vi "LJM logger fill channel setup lists to size.vi"(1 "Default Channel Setup":T1={"Name"=["AIN0", "AIN1", "AIN2", "AIN3", "AIN4", "AIN5", "AIN6", "AIN7", "AIN8", "AIN9", "AIN10", "AIN11", "AIN12", "AIN13", "AIN14", "AIN15", "AIN16", "AIN17", "AIN18", "AIN19", "AIN20", "AIN21", "AIN22", "AIN23", "AIN24", "AIN25", "AIN26", "AIN27", "AIN28", "AIN29", "AIN30", "AIN31", "AIN32", "AIN33", "AIN34", "AIN35", "AIN36", "AIN37", "AIN38", "AIN39", "AIN40", "AIN41", "AIN42", "AIN43", "AIN44", "AIN45", "AIN46", "AIN47", "AIN48", "AIN49", "AIN50", "AIN51", "AIN52", "AIN53", "AIN54", "AIN55", "AIN56", "AIN57", "AIN58", "AIN59", "AIN60", "AIN61", "AIN62", "AIN63", "AIN64", "AIN65", "AIN66", "AIN67", "AIN68", "AIN69", "AIN70", "AIN71", "AIN72", "AIN73", "AIN74", "AIN75", "AIN76", "AIN77", "AIN78", "AIN79", "AIN80", "AIN81", "AIN82", "AIN83", "AIN84", "AIN85", "AIN86", "AIN87", "AIN88", "AIN89", "AIN90", "AIN91", "AIN92", "AIN93", "AIN94", "AIN95", "AIN96", "AIN97", "AIN98", "AIN99"], "", "Scaling Equation"=["y=a", "y=b", "y=c", "y=d", "y=e", "y=f", "y=g", "y=h", "y=i", "y=j", "y=k", "y=l", "y=m", "y=n", "y=o", "y=p", "y=q", "y=r", "y=s", "y=t", "y=u", "y=v", "y=w", "y=x", "y=y", "y=z", "y=a2", "y=b2", "y=c2", "y=d2", "y=e2", "y=f2", "y=g2", "y=h2", "y=i2", "y=j2", "y=k2", "y=l2", "y=m2", "y=n2", "y=o2", "y=p2", "y=q2", "y=r2", "y=s2", "y=t2", "y=u2", "y=v2", "y=w2", "y=x2", "y=y2", "y=z2", "y=a3", "y=b3", "y=c3", "y=d3", "y=e3", "y=f3", "y=g3", "y=h3", "y=i3", "y=j3", "y=k3", "y=l3", "y=m3", "y=n3", "y=o3", "y=p3", "y=q3", "y=r3", "y=s3", "y=t3", "y=u3", "y=v3", "y=w3", "y=x3", "y=y3", "y=z3", "y=a4", "y=b4", "y=c4", "y=d4", "y=e4", "y=f4", "y=g4", "y=h4", "y=i4", "y=j4", "y=k4", "y=l4", "y=m4", "y=n4", "y=o4", "y=p4", "y=q4", "y=r4", "y=s4", "y=t4", "y=u4", "y=v4"], "", "Graph?"=[TRUE, TRUE, TRUE, TRUE, FALSE, FALSE, FALSE, FALSE, FALSE, FALSE, FALSE, FALSE, FALSE, FALSE, FALSE, FALSE]}, 2 "Channel Setup In":T1={"Name"=["AIN0", "AIN1", "AIN2", "AIN3", "AIN4", "AIN5", "AIN6", "AIN7", "AIN8", "AIN9", "AIN10", "AIN11", "AIN12", "AIN13", "AIN14", "AIN15", "AIN16", "AIN17", "AIN18", "AIN19", "AIN20", "AIN21", "AIN22", "AIN23", "AIN24", "AIN25", "AIN26", "AIN27", "AIN28", "AIN29", "AIN30", "AIN31", "AIN32", "AIN33", "AIN34", "AIN35", "AIN36", "AIN37", "AIN38", "AIN39", "AIN40", "AIN41", "AIN42", "AIN43", "AIN44", "AIN45", "AIN46", "AIN47", "AIN48", "AIN49", "AIN50", "AIN51", "AIN52", "AIN53", "AIN54", "AIN55", "AIN56", "AIN57", "AIN58", "AIN59", "AIN60", "AIN61", "AIN62", "AIN63", "AIN64", "AIN65", "AIN66", "AIN67", "AIN68", "AIN69", "AIN70", "AIN71", "AIN72", "AIN73", "AIN74", "AIN75", "AIN76", "AIN77", "AIN78", "AIN79", "AIN80", "AIN81", "AIN82", "AIN83", "AIN84", "AIN85", "AIN86", "AIN87", "AIN88", "AIN89", "AIN90", "AIN91", "AIN92", "AIN93", "AIN94", "AIN95", "AIN96", "AIN97", "AIN98", "AIN99"], "", "Scaling Equation"=["y=a", "y=b", "y=c", "y=d", "y=e", "y=f", "y=g", "y=h", "y=i", "y=j", "y=k", "y=l", "y=m", "y=n", "y=o", "y=p", "y=q", "y=r", "y=s", "y=t", "y=u", "y=v", "y=w", "y=x", "y=y", "y=z", "y=a2", "y=b2", "y=c2", "y=d2", "y=e2", "y=f2", "y=g2", "y=h2", "y=i2", "y=j2", "y=k2", "y=l2", "y=m2", "y=n2", "y=o2", "y=p2", "y=q2", "y=r2", "y=s2", "y=t2", "y=u2", "y=v2", "y=w2", "y=x2", "y=y2", "y=z2", "y=a3", "y=b3", "y=c3", "y=d3", "y=e3", "y=f3", "y=g3", "y=h3", "y=i3", "y=j3", "y=k3", "y=l3", "y=m3", "y=n3", "y=o3", "y=p3", "y=q3", "y=r3", "y=s3", "y=t3", "y=u3", "y=v3", "y=w3", "y=x3", "y=y3", "y=z3", "y=a4", "y=b4", "y=c4", "y=d4", "y=e4", "y=f4", "y=g4", "y=h4", "y=i4", "y=j4", "y=k4", "y=l4", "y=m4", "y=n4", "y=o4", "y=p4", "y=q4", "y=r4", "y=s4", "y=t4", "y=u4", "y=v4"], "", "Graph?"=[TRUE, TRUE, TRUE, TRUE, FALSE, FALSE, FALSE, FALSE, FALSE, FALSE, FALSE, FALSE, FALSE, FALSE, FALSE, FALSE]}) -> (0 "Channel Setup Out":T1={"Name"=["AIN0", "AIN1", "AIN2", "AIN3", "AIN4", "AIN5", "AIN6", "AIN7", "AIN8", "AIN9", "AIN10", "AIN11", "AIN12", "AIN13", "AIN14", "AIN15", "AIN16", "AIN17", "AIN18", "AIN19", "AIN20", "AIN21", "AIN22", "AIN23", "AIN24", "AIN25", "AIN26", "AIN27", "AIN28", "AIN29", "AIN30", "AIN31", "AIN32", "AIN33", "AIN34", "AIN35", "AIN36", "AIN37", "AIN38", "AIN39", "AIN40", "AIN41", "AIN42", "AIN43", "AIN44", "AIN45", "AIN46", "AIN47", "AIN48", "AIN49", "AIN50", "AIN51", "AIN52", "AIN53", "AIN54", "AIN55", "AIN56", "AIN57", "AIN58", "AIN59", "AIN60", "AIN61", "AIN62", "AIN63", "AIN64", "AIN65", "AIN66", "AIN67", "AIN68", "AIN69", "AIN70", "AIN71", "AIN72", "AIN73", "AIN74", "AIN75", "AIN76", "AIN77", "AIN78", "AIN79", "AIN80", "AIN81", "AIN82", "AIN83", "AIN84", "AIN85", "AIN86", "AIN87", "AIN88", "AIN89", "AIN90", "AIN91", "AIN92", "AIN93", "AIN94", "AIN95", "AIN96", "AIN97", "AIN98", "AIN99"], "", "Scaling Equation"=["y=a", "y=b", "y=c", "y=d", "y=e", "y=f", "y=g", "y=h", "y=i", "y=j", "y=k", "y=l", "y=m", "y=n", "y=o", "y=p", "y=q", "y=r", "y=s", "y=t", "y=u", "y=v", "y=w", "y=x", "y=y", "y=z", "y=a2", "y=b2", "y=c2", "y=d2", "y=e2", "y=f2", "y=g2", "y=h2", "y=i2", "y=j2", "y=k2", "y=l2", "y=m2", "y=n2", "y=o2", "y=p2", "y=q2", "y=r2", "y=s2", "y=t2", "y=u2", "y=v2", "y=w2", "y=x2", "y=y2", "y=z2", "y=a3", "y=b3", "y=c3", "y=d3", "y=e3", "y=f3", "y=g3", "y=h3", "y=i3", "y=j3", "y=k3", "y=l3", "y=m3", "y=n3", "y=o3", "y=p3", "y=q3", "y=r3", "y=s3", "y=t3", "y=u3", "y=v3", "y=w3", "y=x3", "y=y3", "y=z3", "y=a4", "y=b4", "y=c4", "y=d4", "y=e4", "y=f4", "y=g4", "y=h4", "y=i4", "y=j4", "y=k4", "y=l4", "y=m4", "y=n4", "y=o4", "y=p4", "y=q4", "y=r4", "y=s4", "y=t4", "y=u4", "y=v4"], "", "Graph?"=[TRUE, TRUE, TRUE, TRUE, FALSE, FALSE, FALSE, FALSE, FALSE, FALSE, FALSE, FALSE, FALSE, FALSE, FALSE, FALSE]})   [LabVIEW 2026]
uses:
  Common Logger Controls/Channel Setup.ctl
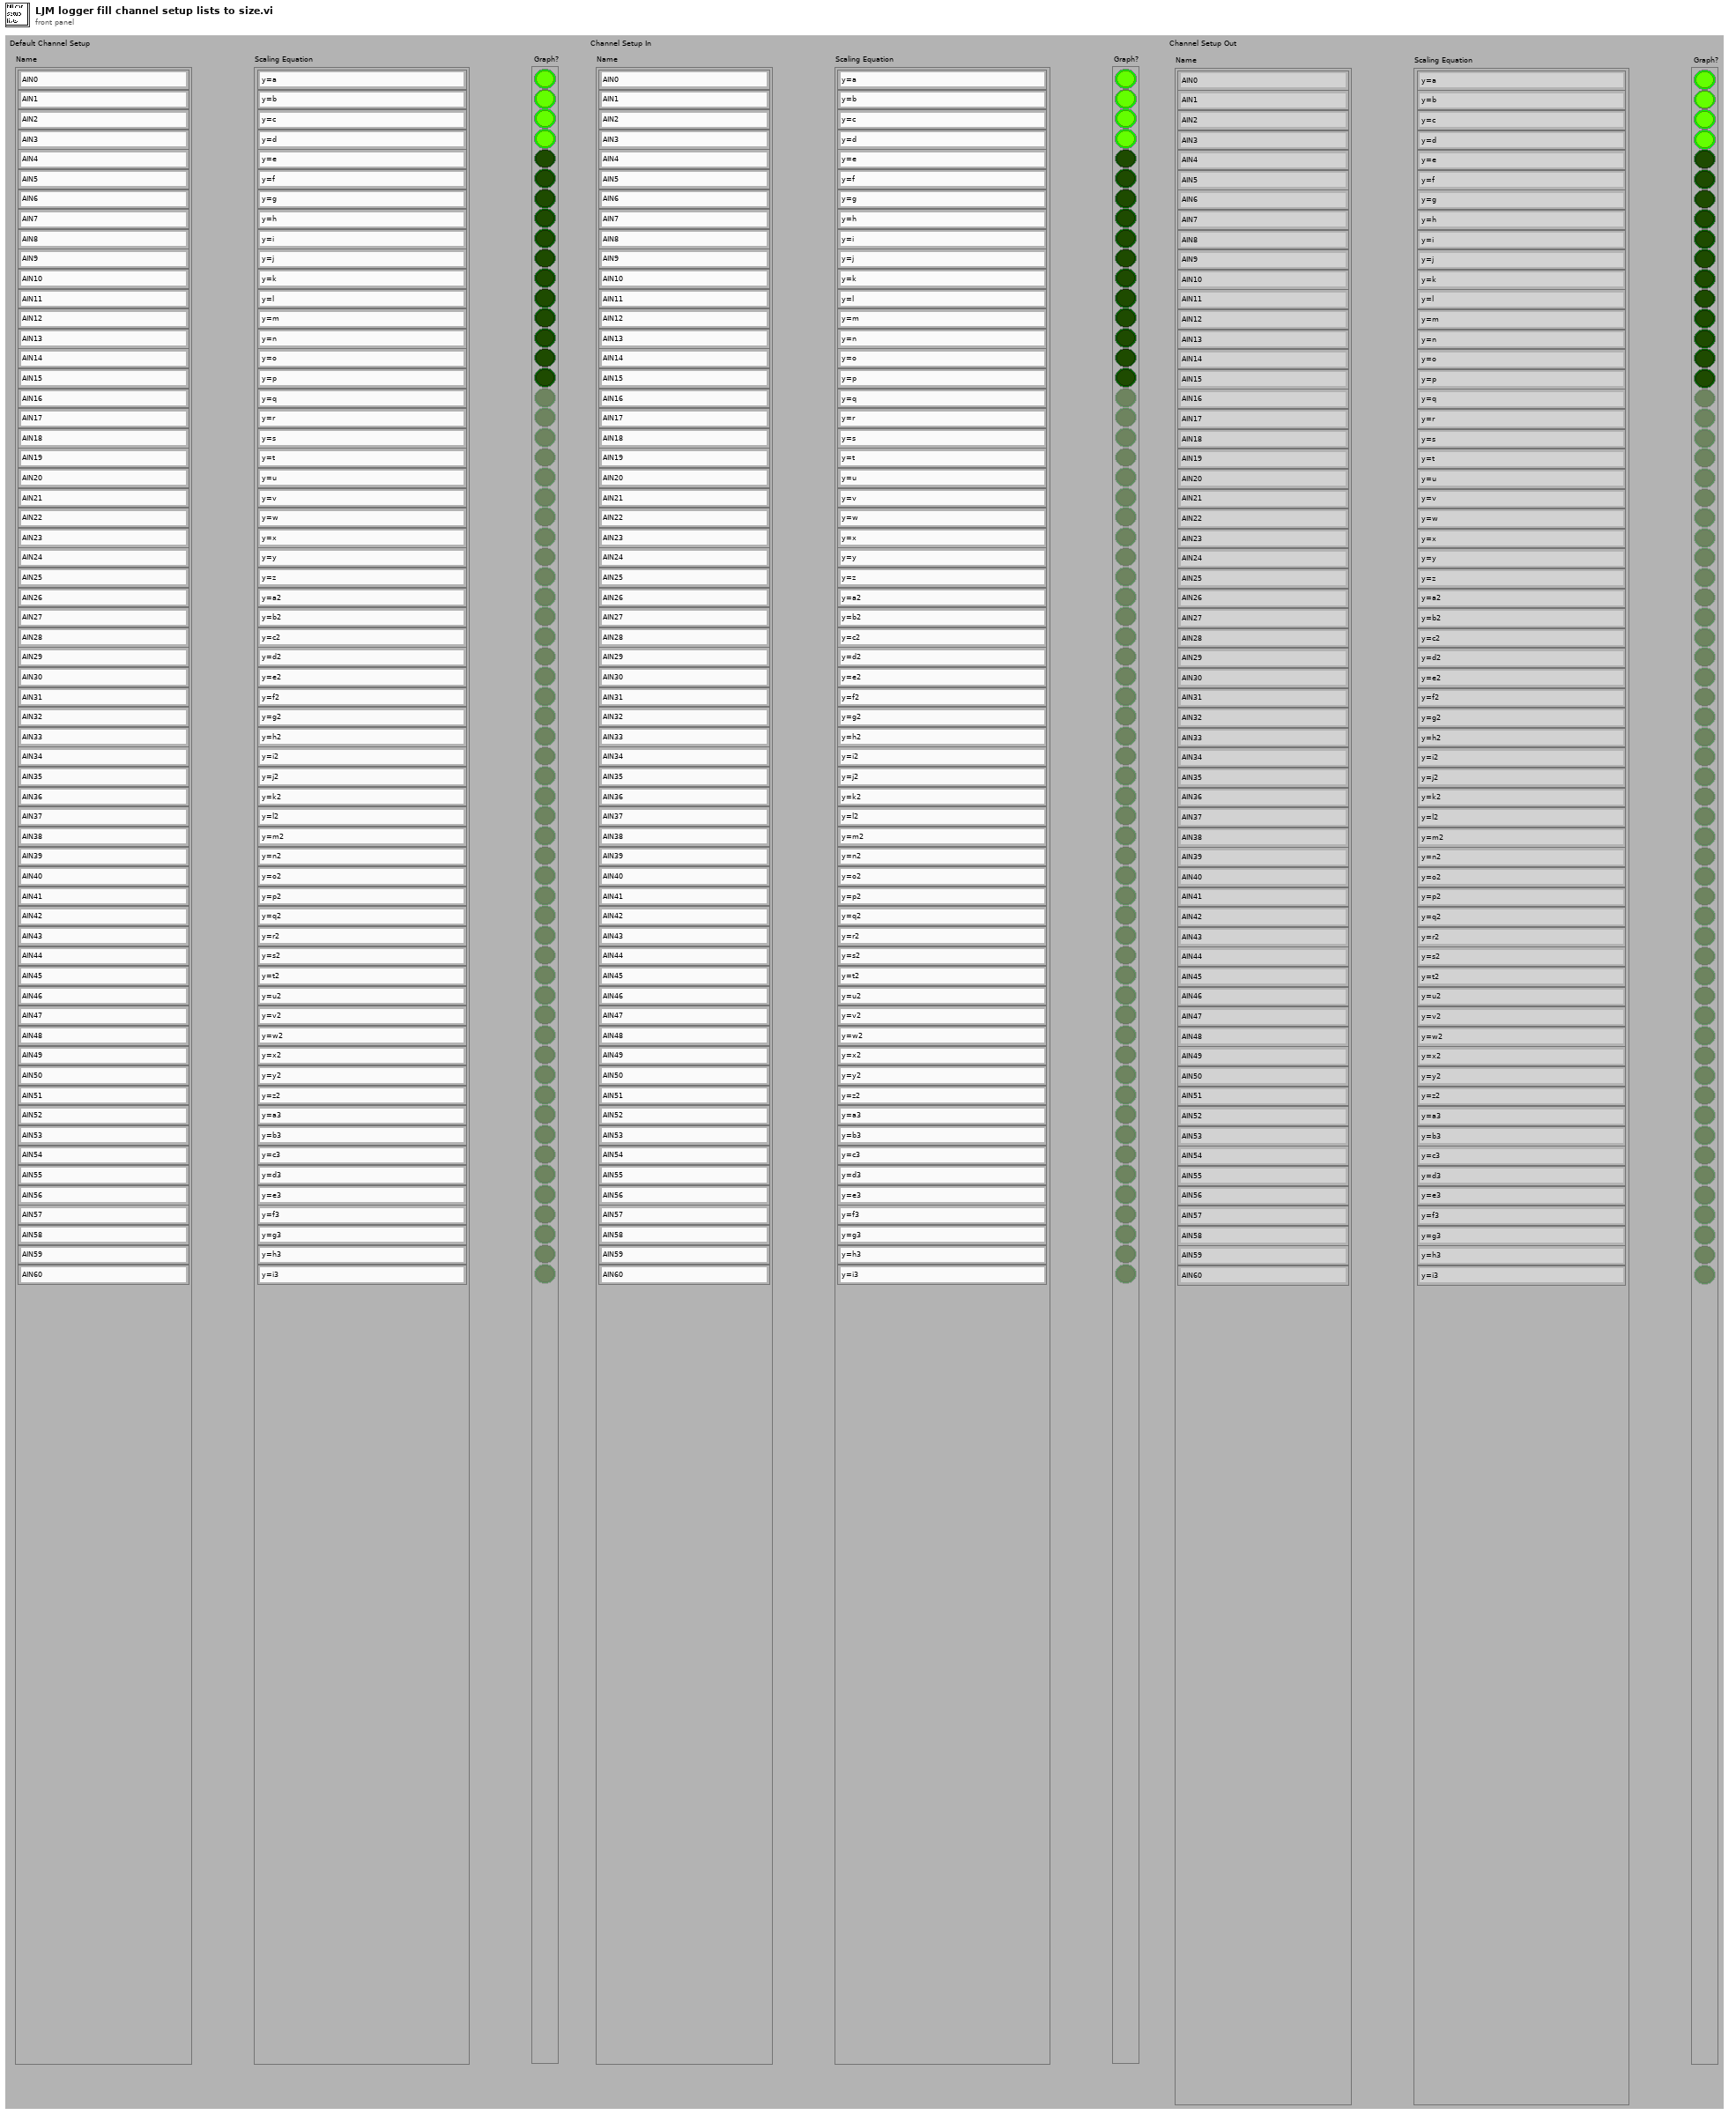
[diagram p1: front panel]
types:
  T1 = typedef "Channel Setup.ctl" = cluster{"Name":string[], string, "Scaling Equation":string[], string, "Graph?":bool[]}
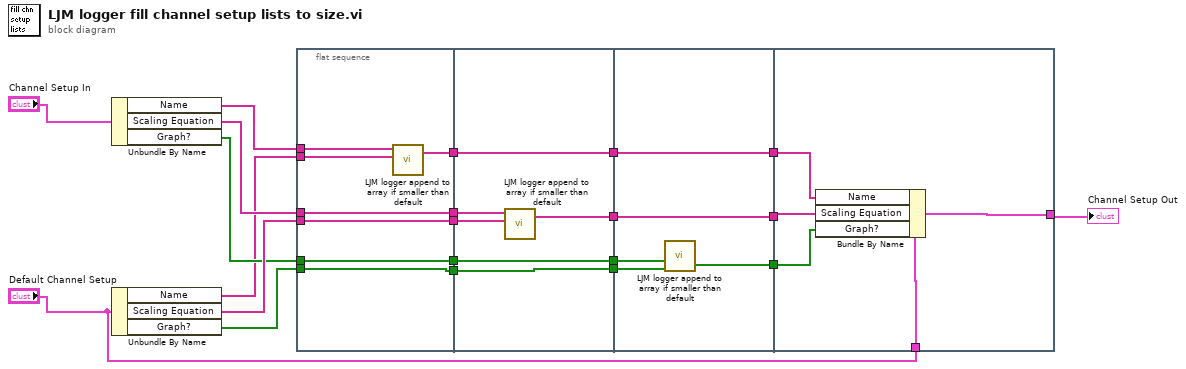
[diagram p0: block diagram]
diagram:
  n1 = Unbundle By Name("Channel Setup In") -> ("Name"=w2:string[], "Scaling Equation"=w19:string[], "Graph?"=w10:bool[])
  n2 = Unbundle By Name("Default Channel Setup") -> ("Name"=w1:string[], "Scaling Equation"=w16:string[], "Graph?"=w11:bool[])
  n3 = flat-sequence {
    tunnel: w2 -> [w28]
    tunnel: w1 -> [w27]
    tunnel: [w26] -> w21
    tunnel: w19 -> [w25]
    tunnel: [w25] -> w18
    tunnel: w16 -> [w24]
    tunnel: [w24] -> w17
    tunnel: w10 -> [w23]
    tunnel: [w23] -> w15
    tunnel: w11 -> [w22]
    tunnel: [w22] -> w13
    tunnel: w21 -> [w34]
    tunnel: [w34] -> w20
    tunnel: w18 -> [w33]
    tunnel: w17 -> [w32]
    tunnel: w15 -> [w31]
    tunnel: [w31] -> w14
    tunnel: w13 -> [w30]
    tunnel: [w30] -> w12
    tunnel: [w29] -> w9
    tunnel: w20 -> [w39]
    tunnel: w14 -> [w38]
    tunnel: w12 -> [w37]
    tunnel: w9 -> [w35]
    tunnel: [w39] -> w8
    tunnel: [w36] -> w7
    tunnel: [w35] -> w6
    tunnel: w8 -> [w44]
    tunnel: w7 -> [w42]
    tunnel: w6 -> [w43]
    tunnel: [w41] -> w4
    tunnel: "Default Channel Setup" -> [w40]
    frame #0 {
      n4 = call "LJM logger append to array if smaller than default.vi"("Default String Array"=w27, "String Array to Check"=w28) -> ("Output String Array"=w26:string[])  [unwired: 2 in, 1 out]
    }
    frame #1 {
      n5 = call "LJM logger append to array if smaller than default.vi"("Default String Array"=w32, "String Array to Check"=w33) -> ("Output String Array"=w29:string[])  [unwired: 2 in, 1 out]
    }
    frame #2 {
      n6 = call "LJM logger append to array if smaller than default.vi"("Default Bool Array"=w37, "Bool Array to Check"=w38) -> ("Output Bool Array"=w36:bool[])  [unwired: 2 in, 1 out]
    }
    frame #3 {
      n7 = Bundle By Name(cluster=w40, "Name"=w44, "Scaling Equation"=w43, "Graph?"=w42) -> (w41:T1)
    }
  }
  "Channel Setup Out" <- w4
